vi "AdorkableWatchDog.vi"() -> ()   [LabVIEW 2014]
panel:
  in  "Stop Button":bool
  out "Functioning?":bool
  out "InstrumentRunning?":bool
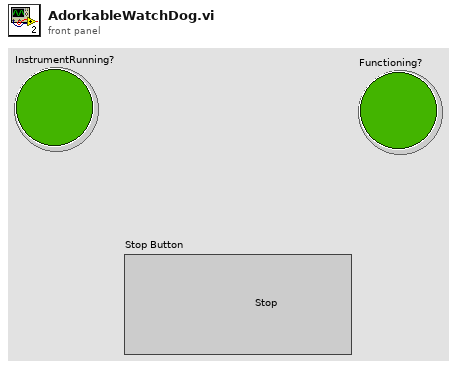
[diagram p1: front panel]
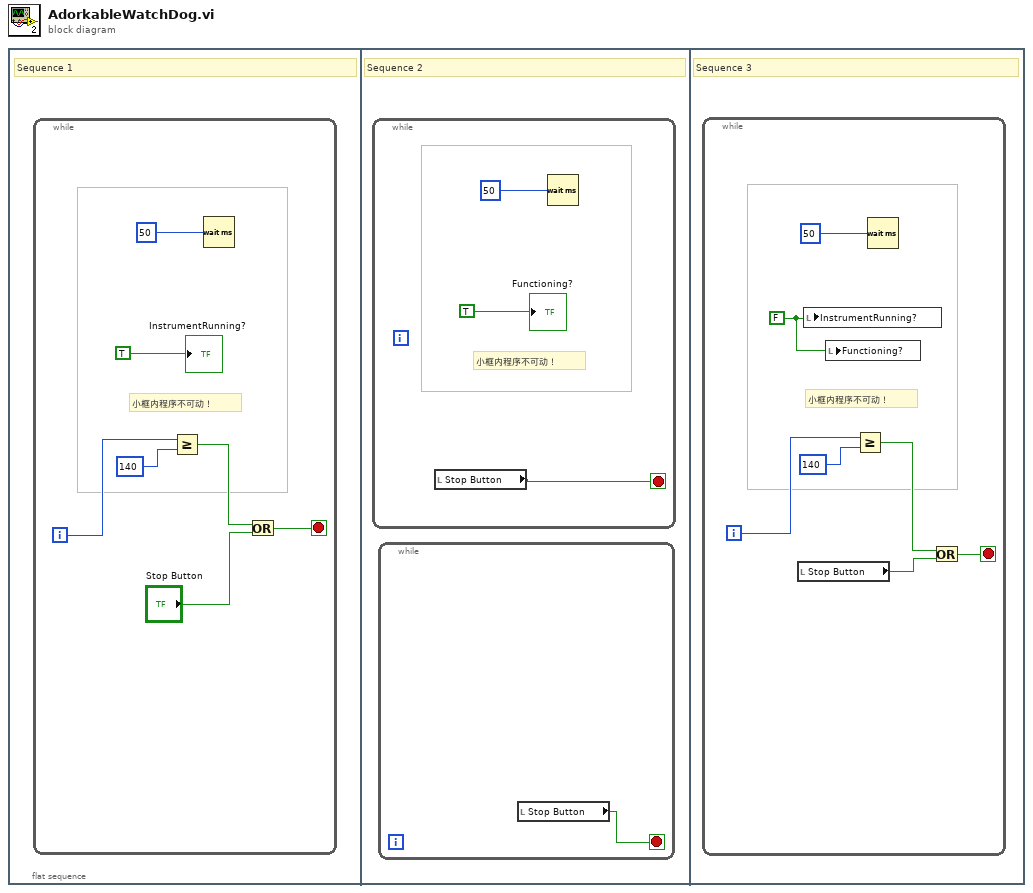
[diagram p0: block diagram]
diagram:
  n1 = flat-sequence {
    frame #0 {
      # "Sequence 1"
      n2 = while {
        i -> [w5]
        stop <- w1 stop-if-true
        # "小框内程序不可动！"
        n3 = Greater Or Equal?(x=w5, y=140) -> (x >= y?=w2:bool)
        n4 = Wait (ms)(milliseconds to wait=u32 50) -> ()  [unwired: 1 out]
        n5 = Or(x=w2, y="Stop Button") -> (x .or. y?=w1:bool)
        "InstrumentRunning?" <- TRUE ("InstrumentRunning?")
      }
    }
    frame #1 {
      # "Sequence 2"
      n6 = while {
        stop <- w9 stop-if-true
        # "小框内程序不可动！"
        n7 = local read "Stop Button"() -> (w9:bool)
        n8 = Wait (ms)(milliseconds to wait=u32 50) -> ()  [unwired: 1 out]
        "Functioning?" <- TRUE ("InstrumentRunning?")
      }
      n9 = while {
        stop <- w8 stop-if-true
        n10 = local read "Stop Button"() -> (w8:bool)
      }
    }
    frame #2 {
      # "Sequence 3"
      n11 = while {
        i -> [w15]
        stop <- w13 stop-if-true
        w17 = FALSE ("InstrumentRunning?")
        # "小框内程序不可动！"
        n12 = local read "Stop Button"() -> (w14:bool)
        n13 = local write "InstrumentRunning?"(w17) -> ()
        n14 = local write "Functioning?"(w17) -> ()
        n15 = Greater Or Equal?(x=w15, y=140) -> (x >= y?=w12:bool)
        n16 = Wait (ms)(milliseconds to wait=u32 50) -> ()  [unwired: 1 out]
        n17 = Or(x=w12, y=w14) -> (x .or. y?=w13:bool)
      }
    }
  }
